vi "sv_Check for Valid Precision.vi"(7 "precision (1)":i16, 8 "error in (no error)":errorcluster) -> (0 "error out":errorcluster)   [LabVIEW 2017, in "SoundVib_Octave_2014 standard.lvlib"]
uses:
  <vilib>/addons/Sound and Vibration/svt_Octave/SoundVib_Octave_2014 standard.lvlib
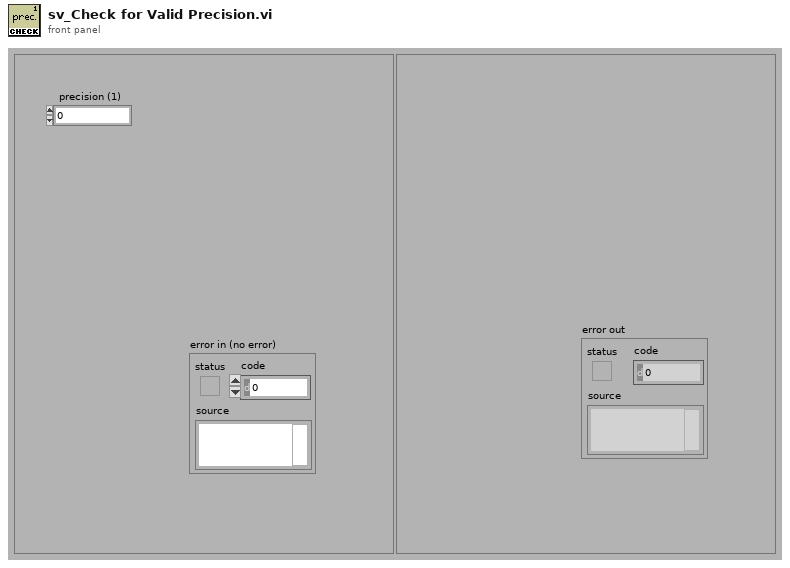
[diagram p1: front panel]
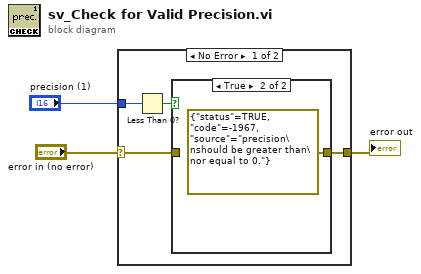
[diagram p0: block diagram]
diagram:
  n1 = case shown="No Error" "error in (no error)" {
    selector: "error in (no error)" -> [w4 w10]
    tunnel: [w7 w10] -> w3
    tunnel: "precision (1)" -> [w5 _]
    frame No Error {
      n2 = Less Than 0?(x=w5) -> (x < 0?=w6:bool)
      n3 = case shown="True" w6 {
        tunnel: w4 -> [w8 _]
        tunnel: [w8 errorcluster {"status"=TRUE, "code"=-1967, "source"="precision\nshould be greater than\nor equal to 0."} ("error IO")] -> w7
        frame False {
        }
        frame True {
        }
      }
    }
    frame Error {
    }
  }
  "error out" <- w3
